vi "DigitalAQ Pines.vi"(8 "error in":errorcluster, 11 "Array":tag[](array[tag])) -> (0 "error out":errorcluster, 3 "Classic DAQmx Task Name":refnum<k21>)   [LabVIEW 2020]
uses:
  <vilib>/DAQmx/create/channels.llb/DAQmx Create Channel (DI-Digital Input).vi
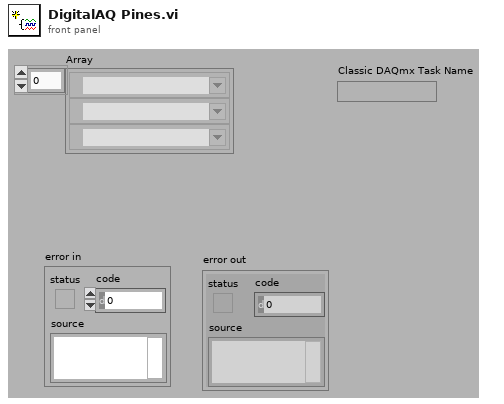
[diagram p1: front panel]
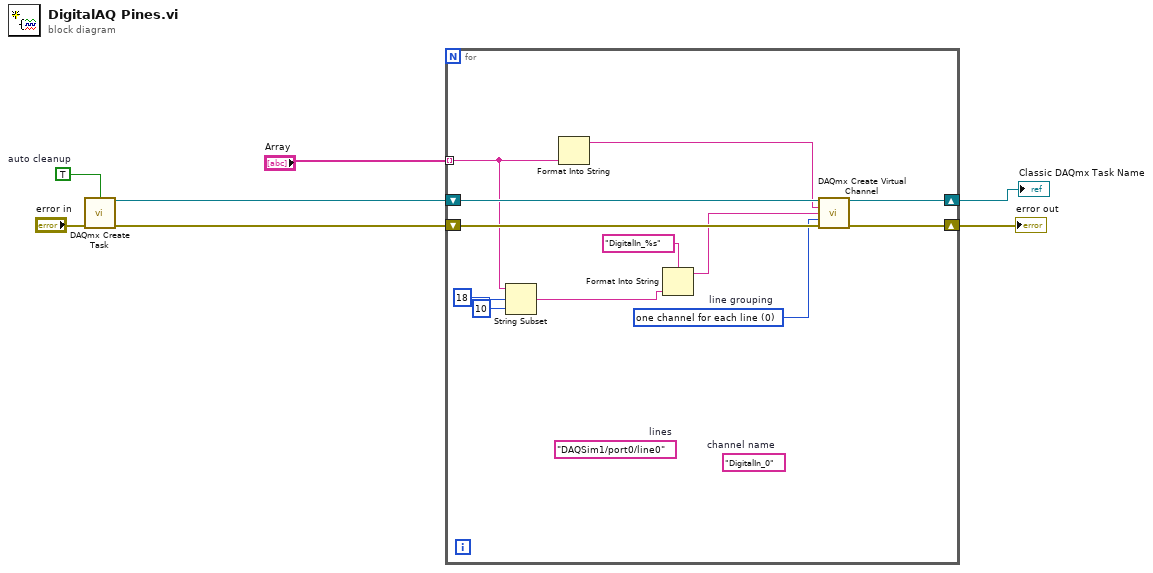
[diagram p0: block diagram]
diagram:
  w5 = TRUE  # auto cleanup
  n1 = call <vilib>:"DAQmx Create Task.vi"("auto cleanup"=w5, "error in"="error in") -> ("task out"=w4:refnum<k21>, "error out"=w6:errorcluster)  [unwired: 12 in]
  n2 = for {
    shift-right: [w16] -> w3
    shift-left: w6 -> [w19]
    shift-right: [w15] -> w2
    shift-left: w4 -> [w18]
    tunnel: "Array" -> [w11] mode=indexing
    w17 = 0 items=["one channel for each line", "one channel for all lines"]  # line grouping
    (unwired) "DigitalIn_0"  # channel name
    (unwired) "DAQSim1/port0/line0"  # lines
    n3 = String Subset(string=w11, offset (0)=18, length (rest)=10 ("length (rest)")) -> (substring=w8:string)
    n4 = Format Into String(w11) -> (resulting string=w12:string)  [unwired: 3 in, 1 out]
    n5 = Format Into String(format string="DigitalIn_%s", w8) -> (resulting string=w13:string)  [unwired: 2 in, 1 out]
    n6 = call-poly <vilib>:"DAQmx Create Virtual Channel.vi"("task in"=w18, "lines"=w12, "name to assign"=w13, "line grouping"=w17, "error in"=w19) -> ("task out"=w15:refnum<k21>, "error out"=w16:errorcluster)  [unwired: 9 in]
  }
  "error out" <- w3
  "Classic DAQmx Task Name" <- w2
